vi "Labview1.vi"() -> ()   [LabVIEW 2014]
uses:
  MT_API/MT_API.lvlib
panel:
  out "当前位置":i32
  out "启动":bool
  in  "确定按钮":bool
  in  "停止":bool
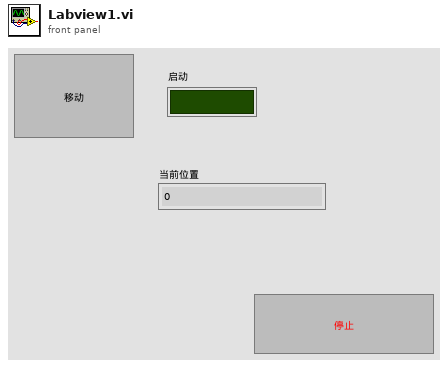
[diagram p1: front panel]
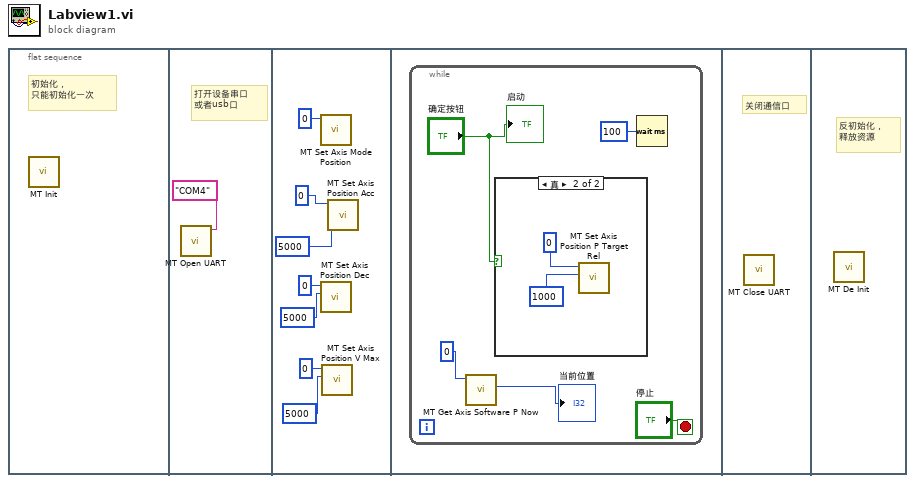
[diagram p0: block diagram]
diagram:
  n1 = flat-sequence {
    frame #0 {
      # "初始化，\n只能初始化一次"
      n2 = call "MT Init.vi"() -> ()  [unwired: 11 in, 1 out]
    }
    frame #1 {
      # "打开设备串口\n或者usb口"
      n3 = call "MT Open UART.vi"("sCOM"="COM4") -> ()  [unwired: 9 in, 2 out]
    }
    frame #2 {
      n4 = call "MT Set Axis Mode Position.vi"("AObj"=u16 0) -> ()  [unwired: 10 in, 1 out]
      n5 = call "MT Set Axis Position Dec.vi"("Value"=5000, "AObj"=u16 0) -> ()  [unwired: 9 in, 1 out]
      n6 = call "MT Set Axis Position V Max.vi"("Value"=5000, "AObj"=u16 0) -> ()  [unwired: 9 in, 1 out]
      n7 = call "MT Set Axis Position Acc.vi"("Value"=5000, "AObj"=u16 0) -> ()  [unwired: 9 in, 1 out]
    }
    frame #3 {
      n8 = while {
        stop <- "停止" stop-if-true
        n9 = call "MT Get Axis Software P Now.vi"("AObj"=u16 0) -> ("pValue out"=→"当前位置":i32)  [unwired: 9 in, 1 out]
        n10 = case shown="真" "确定按钮" {
          frame False {
          }
          frame True {
            n11 = call "MT Set Axis Position P Target Rel.vi"("Value"=1000, "AObj"=u16 0) -> ()  [unwired: 9 in, 1 out]
          }
        }
        n12 = Wait (ms)(milliseconds to wait=u32 100 ("等待时间（毫秒）")) -> ()  [unwired: 1 out]
        "启动" <- "确定按钮"
      }
    }
    frame #4 {
      # "关闭通信口"
      n13 = call "MT Close UART.vi"() -> ()  [unwired: 11 in, 1 out]
    }
    frame #5 {
      # "反初始化，\n释放资源"
      n14 = call "MT De Init.vi"() -> ()  [unwired: 11 in, 1 out]
    }
  }
